vi "Configure Pre DPD Crest Factor Reduction.vi"(0 "Instrument Handle In":refnum<k21>, 1 "Selector String":string, 5 "Pre DPD Crest Factor Reduction Configuration":T2={"Enabled"=1, "Method"=0, "Max Iterations"=10, "Target PAPR (dB)"=8.0, "Shaping Factor"=5.0, "Shaping Threshold (dB)"=-5.0, "Window Type"=7, "Window Length"=10, "Filter Enabled"=0, "Carrier Channels"=[{"Offset (Hz)"=0.0, "Bandwidth (Hz)"=20000000.0}]} {"Carrier Channels"."Bandwidth (Hz)" format="%.2p"; "Carrier Channels"."Offset (Hz)" format="%.2p"; "Filter Enabled" items=["False", "True"]; "Window Type" items=["Flat Top"=1, "Hanning"=2, "Hamming"=3, "Gaussian"=4, "Blackman"=5, "Blackman-Harris"=6, "Kaiser-Bessel"=7]; "Method" items=["Clipping", "Peak Windowing", "Sigmoid"]; "Enabled" items=["False", "True"]}, 7 "Reference Waveform":T1={"Name"="Wfm", "Data"=refnum, "Signal Bandwidth (Hz)"=0.0, "PAPR (dB)"=0.0, "Burst Length (s)"=0.0, "Sample Rate"=0.0, "Burst Start Locations"=[], "Burst Stop Locations"=[], "Idle Duration Present?"=FALSE, "Runtime Scaling"=0.0, "Script"=""} {"Runtime Scaling" format="%#_6p"; "Sample Rate" format="%#_6p"; "Burst Length (s)" format="%#_6p"; "PAPR (dB)" format="%.2f"; "Signal Bandwidth (Hz)" format="%#_6p"}, 11 "error in (no error)":errorcluster) -> (4 "Instrument Handle Out":refnum<k21>, 6 "Pre DPD CFR Waveform":T1={"Name"="Wfm", "Data"=refnum, "Signal Bandwidth (Hz)"=0.0, "PAPR (dB)"=0.0, "Burst Length (s)"=0.0, "Sample Rate"=0.0, "Burst Start Locations"=[], "Burst Stop Locations"=[], "Idle Duration Present?"=FALSE, "Runtime Scaling"=0.0, "Script"=""} {"Runtime Scaling" format="%#_6p"; "Sample Rate" format="%#_6p"; "Burst Length (s)" format="%#_6p"; "PAPR (dB)" format="%.2f"; "Signal Bandwidth (Hz)" format="%#_6p"}, 15 "error out":errorcluster)   [LabVIEW 2019, in "RFmxDPD.lvlib"]
doc: "Configures common pre-DPD CFR settings and applies CFR to the reference waveform, which is returned by the function."
uses:
  RFmxDPD.lvlib
  Common/Waveform.ctl
  Typedefs/Pre DPD Crest Factor Reduction Configuration.ctl
  Typedefs/Pre DPD Crest Factor Reduction Carrier Channel.ctl
  <resource>/objmgr/RFmxSpecAn.rc
  Common/Common.lvlib
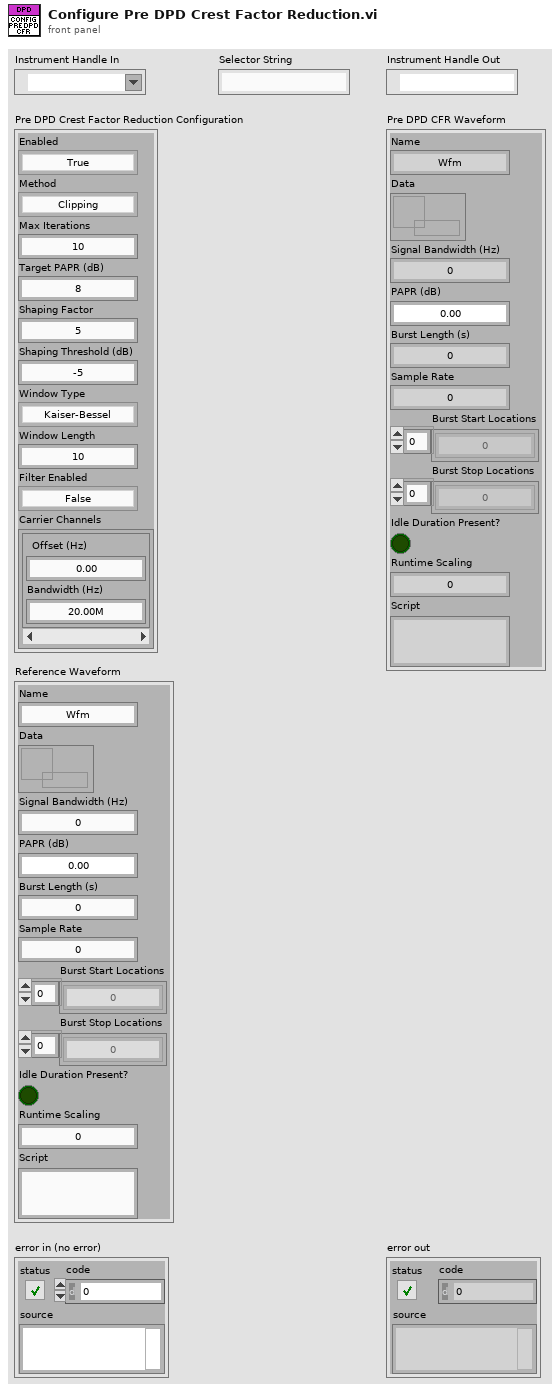
[diagram p1: front panel]
types:
  T1 = typedef "Common.lvlib/Waveform.ctl" = cluster{"Name":string, "Data":refnum<data-value>, "Signal Bandwidth (Hz)":dbl, "PAPR (dB)":dbl, "Burst Length (s)":dbl, "Sample Rate":dbl, "Burst Start Locations":i32[], "Burst Stop Locations":i32[], "Idle Duration Present?":bool, "Runtime Scaling":dbl, "Script":string}
  T2 = typedef "RFmxDPD.lvlib/Pre DPD Crest Factor Reduction Configuration.ctl" = cluster{"Enabled":i32, "Method":i32, "Max Iterations":i32, "Target PAPR (dB)":dbl, "Shaping Factor":dbl, "Shaping Threshold (dB)":dbl, "Window Type":i32, "Window Length":i32, "Filter Enabled":i32, "Carrier Channels":T3[]}
  T3 = typedef "RFmxDPD.lvlib/Pre DPD Crest Factor Reduction Carrier Channel.ctl" = cluster{"Offset (Hz)":dbl, "Bandwidth (Hz)":dbl}
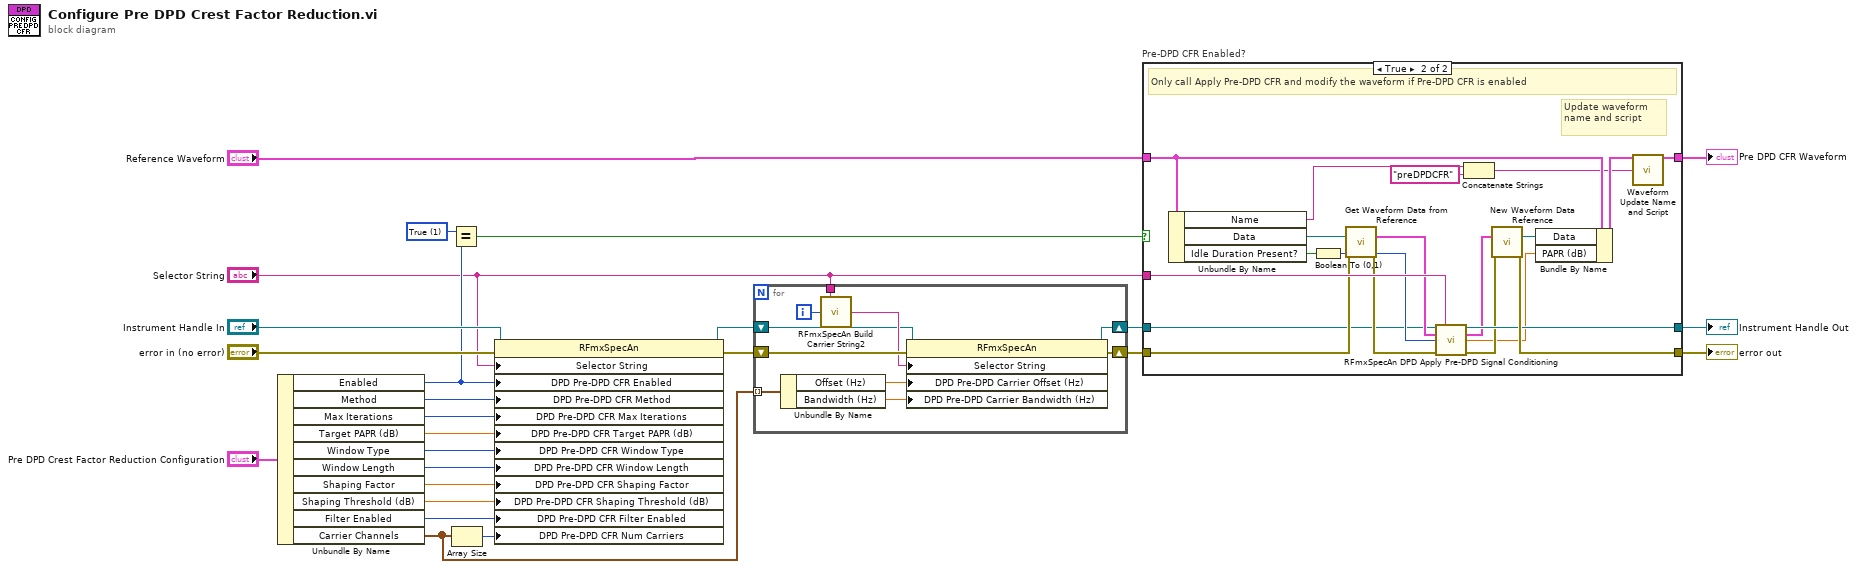
[diagram p0: block diagram]
diagram:
  w9 = 1 items=["False", "True"] ("DPD Pre-DPD CFR Enabled")
  n1 = Unbundle By Name("Pre DPD Crest Factor Reduction Configuration") -> ("Enabled"=w8:i32, "Method"=w19:i32, "Max Iterations"=w18:i32, "Target PAPR (dB)"=w17:dbl, "Window Type"=w16:i32, "Window Length"=w15:i32, "Shaping Factor"=w14:dbl, "Shaping Threshold (dB)"=w13:dbl, "Filter Enabled"=w12:i32, "Carrier Channels"=w11:T3[])
  n2 = Equal?(x=w9, y=w8) -> (x = y?=w1:bool)
  n3 = Array Size(array=w11) -> (size(s)=w3:i32)
  n4 = property class="RFmxSpecAn"(reference="Instrument Handle In", error in="error in (no error)", "Selector String"="Selector String", "DPD Pre-DPD CFR Enabled"=w8, "DPD Pre-DPD CFR Method"=w19, "DPD Pre-DPD CFR Max Iterations"=w18, "DPD Pre-DPD CFR Target PAPR (dB)"=w17, "DPD Pre-DPD CFR Window Type"=w16, "DPD Pre-DPD CFR Window Length"=w15, "DPD Pre-DPD CFR Shaping Factor"=w14, "DPD Pre-DPD CFR Shaping Threshold (dB)"=w13, "DPD Pre-DPD CFR Filter Enabled"=w12, "DPD Pre-DPD CFR Num Carriers"=w3) -> (reference out=w4:refnum<k21>, error out=w6:errorcluster)
  n5 = for {
    shift-right: [w34] -> w5
    shift-left: w6 -> [w35]
    shift-right: [w29] -> w2
    shift-left: w4 -> [w30]
    tunnel: "Selector String" -> [w31]
    tunnel: w11 -> [w28] mode=indexing
    i -> [w33]
    n6 = Unbundle By Name(w28) -> ("Offset (Hz)"=w27:dbl, "Bandwidth (Hz)"=w26:dbl)
    n7 = call <vilib>:"RFmxSpecAn Build Carrier String2.vi"("Selector String"=w31, "Carrier Number"=w33) -> ("Selector String Out"=w32:string)  [unwired: 13 in]
    n8 = property class="RFmxSpecAn"(reference=w30, error in=w35, "Selector String"=w32, "DPD Pre-DPD Carrier Offset (Hz)"=w27, "DPD Pre-DPD Carrier Bandwidth (Hz)"=w26) -> (reference out=w29:refnum<k21>, error out=w34:errorcluster)
  }
  n9 = case "Pre-DPD CFR Enabled?" shown="True" w1 {
    tunnel: [w37 w58] -> w24
    tunnel: "Reference Waveform" -> [w36 w57]
    tunnel: [w36 w56] -> w21
    tunnel: [w38 w55] -> w10
    tunnel: "Selector String" -> [_ w54]
    tunnel: w5 -> [w37 w53]
    tunnel: w2 -> [w38 w39]
    frame False {
    }
    frame True {
      # "Update waveform name and script"
      # "Only call Apply Pre-DPD CFR and modify the waveform if Pre-DPD CFR is enabled"
      n10 = Unbundle By Name(w57) -> ("Name"=w42:string, "Data"=w50:refnum<data-value>, "Idle Duration Present?"=w45:bool)
      n11 = Boolean To (0,1)(Boolean=w45) -> (0, 1=w48:i16)
      n12 = call "Get Waveform Data from Reference.vi"("Waveform Data Reference"=w50, "error in (no error)"=w53) -> ("Waveform Data"=w49:cluster{"t0":dbl, "dt":dbl, "y":csg[]}, "error out"=w52:errorcluster)  [unwired: 12 in]
      n13 = call <vilib>:"RFmxSpecAn DPD Apply Pre-DPD Signal Conditioning.vi"("Instrument Handle In"=w39, "Selector String"=w54, "Waveform In"=w49, "Idle Duration Present"=w48, "error in (no error)"=w52) -> ("Instrument Handle Out"=w55:refnum<k21>, "Waveform Out"=w46:cluster{"x0":dbl, "dx":dbl, "y":csg[]}, "PAPR (dB)"=w44:dbl, "error out"=w51:errorcluster)  [unwired: 7 in]
      n14 = Concatenate Strings(w42, "preDPDCFR" ("string")) -> (w40:string)
      n15 = call "New Waveform Data Reference.vi"("Waveform Data"=w46, "error in (no error)"=w51) -> ("Waveform Data Reference"=w43:refnum<data-value>, "error out"=w58:errorcluster)  [unwired: 12 in]
      n16 = Bundle By Name(cluster=w57, "Data"=w43, "PAPR (dB)"=w44) -> (w41:T1)
      n17 = call "Waveform Update Name and Script.vi"("Waveform in"=w41, "New Waveform Name"=w40) -> ("Waveform out"=w56:T1)  [unwired: 13 in]
    }
  }
  "error out" <- w24
  "Instrument Handle Out" <- w10
  "Pre DPD CFR Waveform" <- w21
